vi "stage step to next field globals.vi"() -> ()   [LabVIEW 2011]
panel:
  in  "# Fields across y":i8(slide)=3 min=1 max=10 step=1 scale=0.0..10.0
  in  "# Fields across x":i8(slide)=3 min=1 max=10 step=1 scale=0.0..10.0
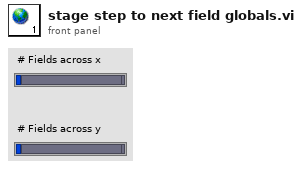
[diagram p1: front panel]
diagram:
